vi "Dut Connect.vi"(0 "MTK7615 in":refnum<class "MTK7615.lvclass">, 5 "Auto Interface":bool=TRUE, 11 "error in (no error)":errorcluster) -> (4 "MTK7615 out":refnum<class "MTK7615.lvclass">, 15 "error out":errorcluster)   [LabVIEW 2015, in "MTK7615.lvlib" / "MTK7615.lvclass"]
uses:
  MTK7615.lvclass
  D:/My Projects/WTS/MTK7615/MTK7615/TelnetDUTControl/TypeDef/niDCT_TELNET_Priv.ctl
  CommLib/Utility/telnet/telnet.llb/Telnet Session.ctl
  CommLib/Includes/niDTS Comm String INC Handle.ctl
  CommLib/Objects/String_class/niDTS Comm String.lvclass
  CommLib/Includes/niDTS Comm Telnet INC Handle.ctl
  CommLib/Objects/Telnet_class/niDTS Comm Telnet.lvclass
  MTK7615.lvclass/MTK7615.ctl
  Framework/Comm/Objects/BASE_class/niDTS Comm.lvclass
  CommLib/niDTS CommLib.lvlib
  Framework/niDTS Framework.lvlib
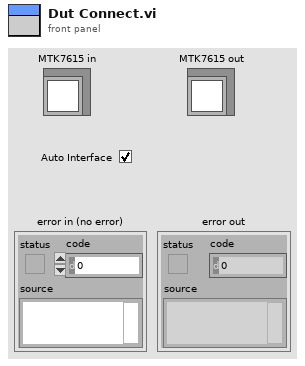
[diagram p1: front panel]
types:
  T1 = typedef "niDTS CommLib.lvlib/niDTS Comm Telnet INC Handle.ctl" = refnum<data-value>
  T2 = typedef "niDTS CommLib.lvlib/niDTS Comm String INC Handle.ctl" = refnum<data-value>
  T3 = typedef "niDCT_TELNET_Priv.ctl" = cluster{"Name":string, "Telnet":T4, "LogInfo":cluster{"DutIP":string, "LocalIP":string, "LocalPort":u16, "UserName?":bool, "UsrNamePrompt":string, "UserName":string, "PwdPrompt":string, "Pwd":string, "CliLogin?":bool, "CLIPrompt":string, "Shell":string}, "CMDPrompt":string, "ACKTimeout":i32, "RebootTO":i32, "2G_ID":string, "2G_CmdHead":string, "5G_ID":string, "5G_CmdHead":string, "2chip?":bool, "2G5Gsel?":bool}
  T4 = typedef "Telnet Session.ctl" = refnum<k1>
  T5 = typedef "niDTS Framework.lvlib/niDTS Comm INC Handle.ctl" = refnum<data-value>
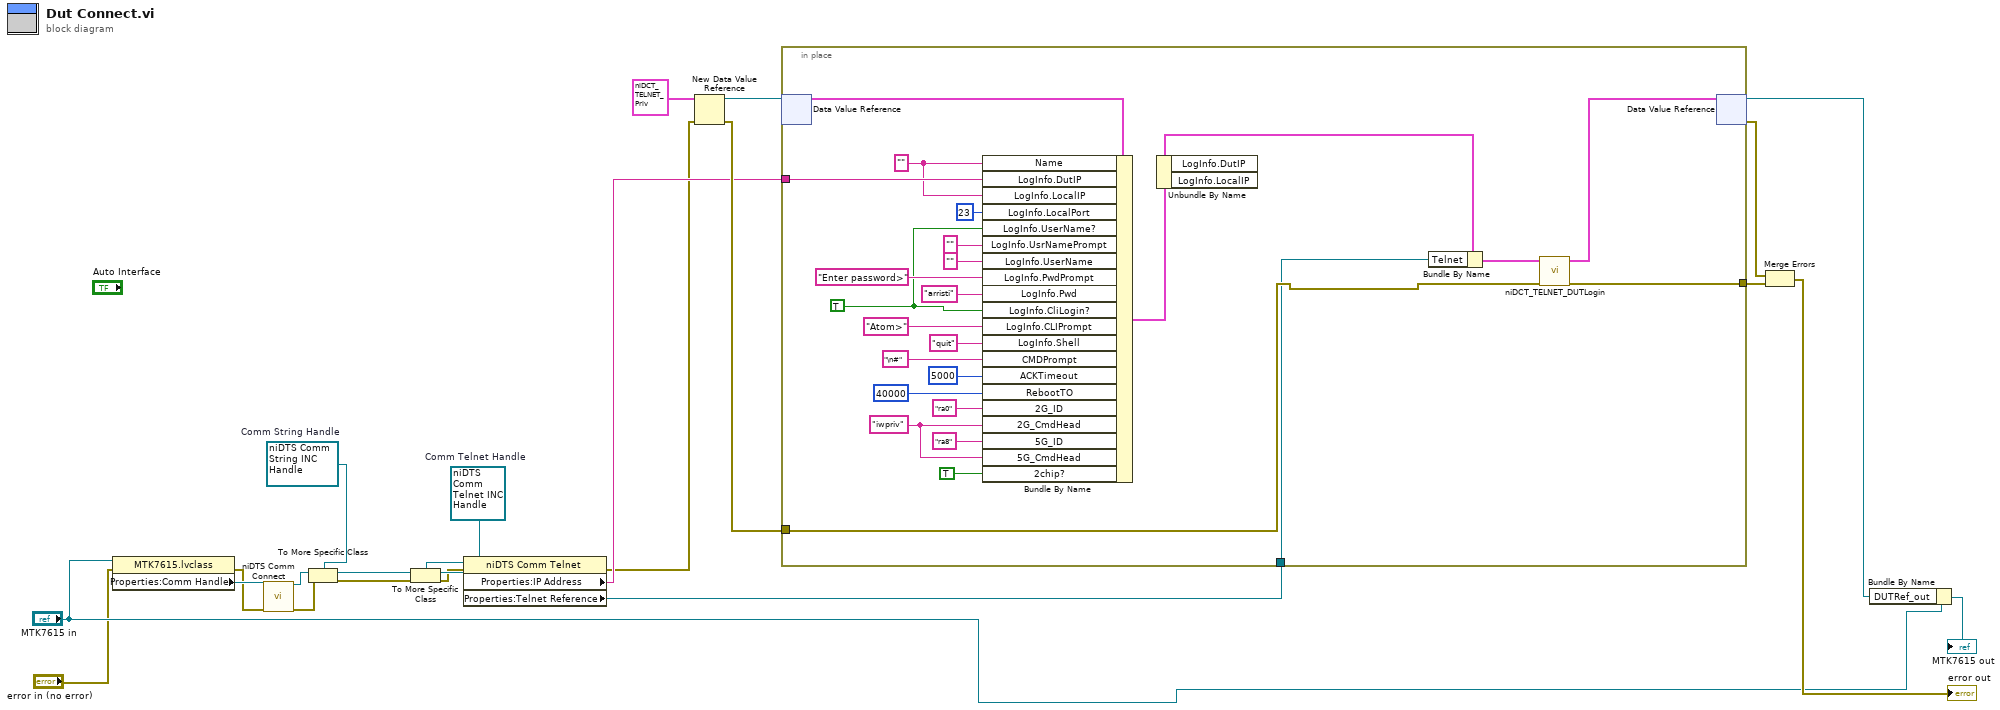
[diagram p0: block diagram]
diagram:
  w16 = T1 refnum  # Comm Telnet Handle
  w18 = T2 refnum  # Comm String Handle
  n1 = property class="MTK7615.lvclass"(reference="MTK7615 in", error in="error in (no error)") -> (error out=w5:errorcluster, "Properties:Comm Handle"=w8:T5)  [unwired: 1 out]
  n2 = call "niDTS Comm Connect.vi"("Comm Handle In"=w8, "error in (no error)"=w5) -> ("Comm Handle"=w7:T5, "error out"=w4:errorcluster)  [unwired: 12 in]
  n3 = To More Specific Class(target class=w18, reference=w7, error in=w4) -> (specific class reference=w17:T2, error out=w3:errorcluster)
  n4 = To More Specific Class(target class=w16, reference=w17, error in=w3) -> (specific class reference=w15:T1, error out=w2:errorcluster)
  n5 = property class="niDTS Comm Telnet"(reference=w15, error in=w2) -> (error out=w1:errorcluster, "Properties:IP Address"=w14:string, "Properties:Telnet Reference"=w13:T4)  [unwired: 1 out]
  n6 = New Data Value Reference(data value=T3 {"Name"="", "Telnet"=refnum, "LogInfo"={"DutIP"="192.168.1.1", "LocalIP"="192.168.1.100", "LocalPort"=23, "UserName?"=TRUE, "UsrNamePrompt"="", "UserName"="admin", "PwdPrompt"="", "Pwd"="admin", "CliLogin?"=TRUE, "CLIPrompt"=">", "Shell"="sh"}, "CMDPrompt"="#", "ACKTimeout"=5000, "RebootTO"=40000, "2G_ID"="admin", "2G_CmdHead"="admin", "5G_ID"="admin", "5G_CmdHead"="admin", "2chip?"=TRUE, "2G5Gsel?"=TRUE}, error in=w1) -> (data value reference=w20:refnum<data-value>, error out=w19:errorcluster)
  n7 = in-place {
    in-place-border: w19 -> [w29]
    in-place-border: [w34] -> w22
    in-place-border: w14 -> [w28]
    in-place-border: w13 -> [w26]
    w24 = TRUE ("LogInfo.CliLogin?")
    w27 = "" ("Name")
    w31 = "iwpriv" ("2G_CmdHead")
    n8 = in-place-dvr #1(w20) -> (w47:T3)  [unwired: 1 out]
    n9 = Bundle By Name(cluster=w47, "Name"=w27, "LogInfo.DutIP"=w28, "LogInfo.LocalIP"=w27, "LogInfo.LocalPort"=u16 23, "LogInfo.UserName?"=w24, "LogInfo.UsrNamePrompt"="", "LogInfo.UserName"="", "LogInfo.PwdPrompt"="Enter password>", "LogInfo.Pwd"="arristi", "LogInfo.CliLogin?"=w24, "LogInfo.CLIPrompt"="Atom>", "LogInfo.Shell"="quit", "CMDPrompt"="\n#", "ACKTimeout"=5000, "RebootTO"=40000, "2G_ID"="ra0", "2G_CmdHead"=w31, "5G_ID"="ra8", "5G_CmdHead"=w31, "2chip?"=TRUE) -> (w37:T3)
    n10 = Unbundle By Name(w37) -> ()  [unwired: 2 out]
    n11 = Bundle By Name(cluster=w37, "Telnet"=w26) -> (w36:T3)
    n12 = call "niDCT_TELNET_DUTLogin.vi"("error in (no error)"=w29, "DUTPrivData"=w36) -> ("error out"=w34:errorcluster, "DUTPrivDataOut"=w35:T3)  [unwired: 8 in]
    n13 = in-place-dvr #1(w35) -> (w10:refnum<data-value>, w23:errorcluster)
  }
  n14 = Merge Errors(w23, w22) -> (→"error out":errorcluster)
  n15 = Bundle By Name(cluster="MTK7615 in", "DUTRef_out"=w10) -> (→"MTK7615 out":refnum<class "MTK7615.lvclass">)
